vi "newcal.vi"() -> ()   [LabVIEW 2015]
panel:
  out "XY Graph":cluster{"X":dbl, "Y":dbl}[](graph)
  in  "Numeric 2":dbl
  out "Waveform Chart":dbl(graph)
  in  "Slide":dbl(slide) scale=0.0..10.0
  in  "Numeric":dbl
  in  "stop":bool
  out "display":dbl format="%#_15g"
  in  "Cluster":T1
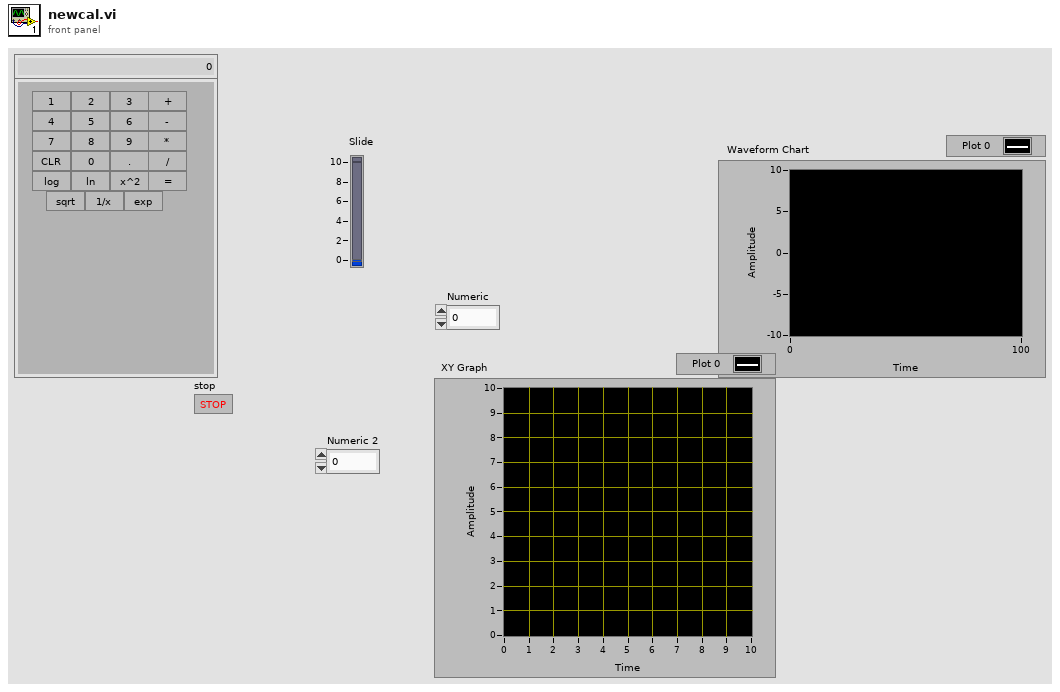
[diagram p1: front panel]
types:
  T1 = cluster{"2":bool, "3":bool, "4":bool, "5":bool, "6":bool, "7":bool, "8":bool, "9":bool, "0":bool, ".":bool, "1":bool, "add":bool, "sub":bool, "devide":bool, "multi":bool, "result 2":bool, "clear":bool, " square":bool, " log":bool, " ln":bool, "sqrt":bool, "1/x":bool, " exp":bool}
  T2 = cluster{" square":bool, " log":bool, " ln":bool, "sqrt":bool, "1/x":bool, " exp":bool}
  T3 = cluster{"add":bool, "sub":bool, "devide":bool, "multi":bool, "result 2":bool}
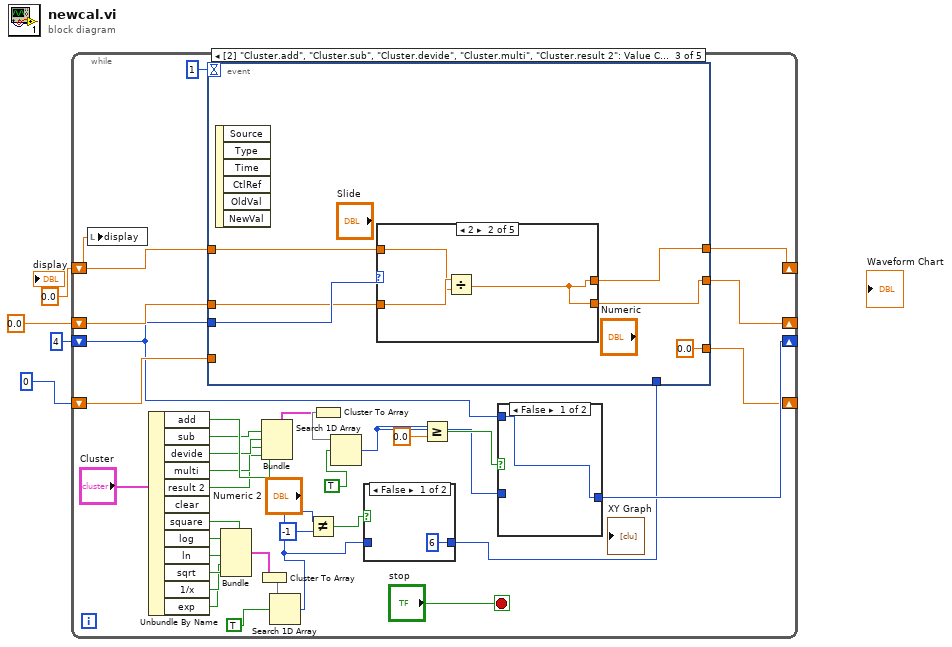
[diagram p0: block diagram]
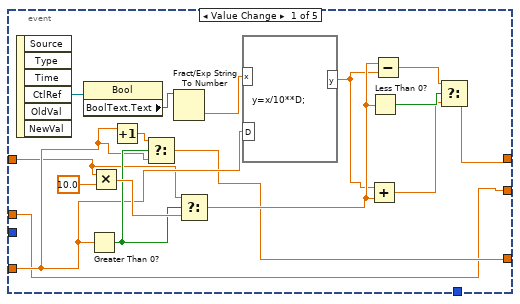
[diagram p4: hidden frame]
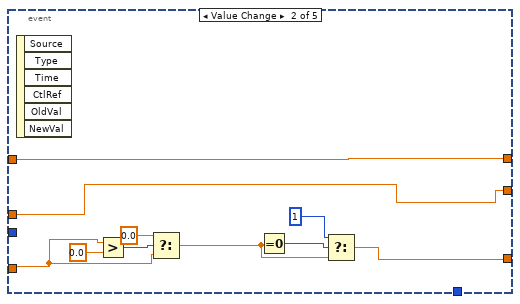
[diagram p5: hidden frame]
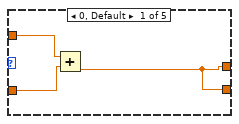
[diagram p6: hidden frame]
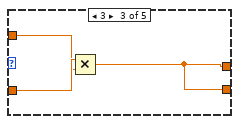
[diagram p7: hidden frame]
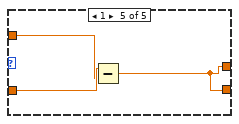
[diagram p9: hidden frame]
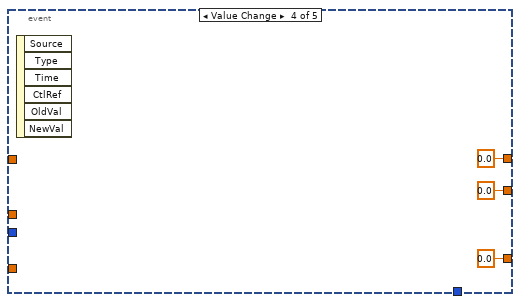
[diagram p10: hidden frame]
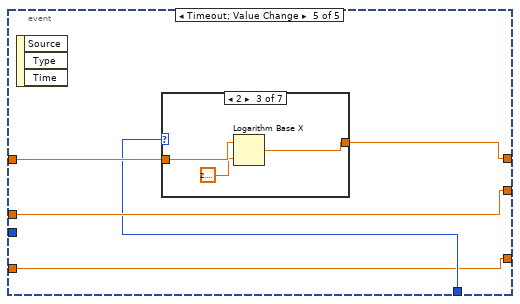
[diagram p11: hidden frame]
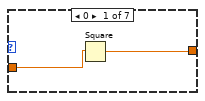
[diagram p12: hidden frame]
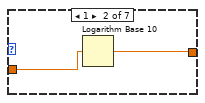
[diagram p13: hidden frame]
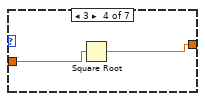
[diagram p14: hidden frame]
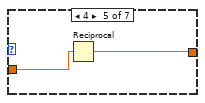
[diagram p15: hidden frame]
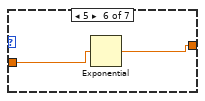
[diagram p16: hidden frame]
diagram:
  n1 = while {
    shift-right: [w39] -> _
    shift-left: 0.0 -> [w38]
    shift-right: [w5] -> _
    shift-left: 0 -> [w36]
    shift-right: [w22] -> _
    shift-left: 4 ("index of element") -> [w21]
    shift-right: [w35] -> _
    shift-left: 0.0 -> [w34]
    stop <- "stop" stop-if-true
    n2 = local write "display"(w38) -> ()
    n3 = Unbundle By Name("Cluster") -> ("add"=w28:bool, "sub"=w27:bool, "devide"=w26:bool, "multi"=w25:bool, "result 2"=w24:bool, "square"=w20:bool, "log"=w19:bool, "ln"=w18:bool, "sqrt"=w17:bool, "1/x"=w7:bool, "exp"=w6:bool)  [unwired: 1 out]
    n4 = Bundle("square"=w20, "log"=w19, "ln"=w18, "sqrt"=w17, "1/x"=w7, "exp"=w6) -> (w16:T2)  [unwired: 1 in]
    n5 = Cluster To Array(cluster=w16) -> (array=w14:bool[])
    n6 = Bundle("add"=w28, "sub"=w27, "devide"=w26, "multi"=w25, "result 2"=w24) -> (w32:T3)  [unwired: 1 in]
    n7 = Search 1D Array(1D array=w14, element=TRUE) -> (index of element=w10:i32)  [unwired: 1 in]
    n8 = Not Equal?(x=w10, y=-1) -> (x != y?=w11:bool)
    n9 = Cluster To Array(cluster=w32) -> (array=w33:bool[])
    n10 = Search 1D Array(1D array=w33, element=TRUE) -> (index of element=w23:i32)  [unwired: 1 in]
    n11 = case shown="False" w11 {
      tunnel: w10 -> [_ w41]
      tunnel: [6 ("index of element") w41] -> w9
      frame False {
      }
      frame True {
      }
    }
    n12 = event shown="[2] \"Cluster.add\", \"Cluster.sub\", \"Cluster.devide\", \"Cluster.multi\", \"Cluster.result 2\": Value Change" {
      selector: _ -> [_ _ _ _ _]
      dyn-events: _ -> [_ _ _ _ _]
      timeout: 1 -> [_ _ _ _ _]
      tunnel: [w55 w70 w72 0.0 w95] -> w39
      tunnel: w38 -> [w44 w70 w75 _ w96]
      tunnel: w36 -> [w47 w61 _ _ w93]
      tunnel: [w46 w69 0.0 ("t") 0.0 ("t") w93] -> w5
      tunnel: w34 -> [w45 w66 w73 _ w97]
      tunnel: [w45 w66 w74 0.0 w97] -> w35
      tunnel: w21 -> [_ _ w76 _ _]
      tunnel: w9 -> [_ _ _ _ w94]
      event "Cluster.1", "Cluster.2", "Cluster.3", "Cluster.4", "Cluster.5", "Cluster.6", "Cluster.7", "Cluster.8", "Cluster.9", "Cluster.0": Value Change {
        n13 = event-data() -> ("CtlRef"=w60:refnum<vi>)  [unwired: 1 in, 5 out]
        n14 = property class="Bool"(reference=w60) -> ("BoolText.Text"=w59:string)  [unwired: 1 in, 2 out]
        n15 = Greater Than 0?(x=w47) -> (x > 0?=w49:bool)
        n16 = Multiply(x=w44, y=10.0) -> (x*y=w52:dbl)
        n17 = Increment(x=w47) -> (x+1=w48:dbl)
        n18 = Select(t=w48, s=w49, f=w47) -> (s? t:f=w46:dbl)
        n19 = Fract/Exp String To Number(string=w59) -> (number=w51:dbl)  [unwired: 3 in, 1 out]
        n20 = Select(t=w44, s=w49, f=w52) -> (s? t:f=w53:dbl)
        n21 = formula code="y=x/10**D;"("x"=w51, "D"=w47) -> ("y"=w50:dbl)
        n22 = Add(x=w50, y=w53) -> (x+y=w56:dbl)
        n23 = Less Than 0?(x=w53) -> (x < 0?=w57:bool)
        n24 = Subtract(x=w53, y=w50) -> (x-y=w54:dbl)
        n25 = Select(t=w54, s=w57, f=w56) -> (s? t:f=w55:dbl)
      }
      event "Cluster..": Value Change {
        n26 = event-data() -> ()  [unwired: 1 in, 6 out]
        n27 = Greater?(x=w61, y=0.0) -> (0:w64:bool)
        n28 = Select(t=0.0, s=w64, f=w61) -> (s? t:f=w62:dbl)
        n29 = Equal To 0?(x=w62) -> (x = 0?=w67:bool)
        n30 = Select(t=1, s=w67, f=w62) -> (s? t:f=w69:dbl)
      }
      event "Cluster.add", "Cluster.sub", "Cluster.devide", "Cluster.multi", "Cluster.result 2": Value Change {
        n31 = event-data() -> ()  [unwired: 1 in, 6 out]
        n32 = case shown="2" w76 {
          tunnel: w75 -> [w79 w81 w84 w86 w88]
          tunnel: [w77 w80 w83 w86 w87] -> w74
          tunnel: w73 -> [w78 w82 w85 _ w89]
          tunnel: [w77 w80 w83 _ w87] -> w72
          frame 0, Default {
            n33 = Add(x=w79, y=w78) -> (x+y=w77:dbl)
          }
          frame 2 {
            n34 = Divide(x=w82, y=w81) -> (x/y=w80:dbl)
          }
          frame 3 {
            n35 = Multiply(x=w85, y=w84) -> (x*y=w83:dbl)
          }
          frame 4 {
          }
          frame 1 {
            n36 = Subtract(x=w89, y=w88) -> (x-y=w87:dbl)
          }
        }
      }
      event "Cluster.clear": Value Change {
        n37 = event-data() -> ()  [unwired: 1 in, 6 out]
      }
      event Timeout; "Cluster.log", "Cluster.ln", "Cluster.sqrt", "Cluster.square", "Cluster.1/x", "Cluster.exp": Value Change {
        n38 = event-data() -> ()  [unwired: 1 in, 3 out]
        n39 = case shown="2" w94 {
          tunnel: w96 -> [w99 w101 w104 w106 w108 w110 w111]
          tunnel: [w98 w100 w102 w105 w107 w109 w111] -> w95
          frame 0 {
            n40 = Square(x=w99) -> (x^2=w98:dbl)
          }
          frame 1 {
            n41 = Logarithm Base 10(1:w101) -> (0:w100:dbl)
          }
          frame 2 {
            n42 = Logarithm Base X(1:2.718281828459045, 2:w104) -> (0:w102:dbl)
          }
          frame 3 {
            n43 = Square Root(x=w106) -> (sqrt(x)=w105:dbl)
          }
          frame 4 {
            n44 = Reciprocal(x=w108) -> (1/x=w107:dbl)
          }
          frame 5 {
            n45 = Exponential(1:w110) -> (0:w109:dbl)
          }
          frame 6, Default {
          }
        }
      }
    }
    n46 = Greater Or Equal?(x=w23, y=0.0) -> (x >= y?=w30:bool)
    n47 = case shown="False" w30 {
      tunnel: [w42 w43] -> w22
      tunnel: w23 -> [_ w43]
      tunnel: w21 -> [w42 _]
      frame False {
      }
      frame True {
      }
    }
  }
